vi "Continuous ERD Write_Stop.vi"(0 "Queue Name":string="ERD Write 1", 11 "Error In":errorcluster) -> (15 "Error Out":errorcluster)   [LabVIEW 2016]
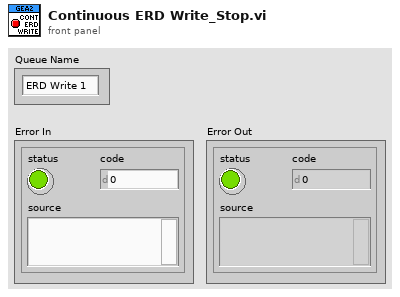
[diagram p1: front panel]
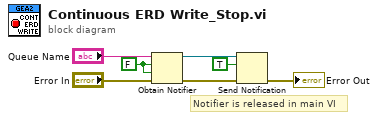
[diagram p0: block diagram]
diagram:
  w5 = FALSE ("create if not found? (T)")
  # "Notifier is released in main VI"
  n1 = Obtain Notifier(name (unnamed)="Queue Name", notification data type=w5, create if not found? (T)=w5, error in (no error)="Error In") -> (notifier out=w4:refnum<notifier>, error out=w2:errorcluster)  [unwired: 1 out]
  n2 = Send Notification(notification=TRUE, notifier=w4, error in (no error)=w2) -> (error out=→"Error Out":errorcluster)  [unwired: 1 out]
